vi "Vehicle Dynamics.vi"(9 "dt":sgl=1.0 format="%0.2f", 10 "Brake Force (N)":sgl, 11 "Transmission Output Torque (N-m)":sgl) -> (1 "Transmission Output Speed (rad/s)":sgl, 2 "Vehicle Speed (miles per hour)":sgl)   [LabVIEW 2016, in "NI-PCG Vehicle Model.lvlib"]
uses:
  NI-PCG Vehicle Model.lvlib
  Globals/Parameters.vi
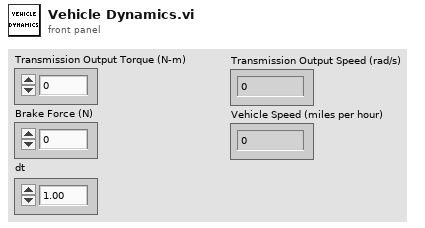
[diagram p1: front panel]
types:
  T1 = typedef "NI-PCG Vehicle Model.lvlib/Engine Parameters.ctl" = cluster{"Ambient Parameters":cluster{"Temperature (K)":sgl, "Pressure (Pa)":sgl}, "Air Parameters":cluster{"R (Ideal Gas Constant)":sgl, "Molecular Weight":sgl, "Cp (Specific Heat Constant)":sgl, "Density (kg/m^3)":sgl, "Stoichiometric A/F Ratio":sgl}, "Engine Geometry Parameters":cluster{"Cylinder Volume (l)":sgl, "J (Rotational Moment of Inertia)":sgl, "Minimuim Engine Speed":sgl, "Maximum Engine Speed":sgl, "Intake Manifold Volume (l)":sgl}, "Volumetric Efficiency Map":cluster{"MAP":sgl[], "RPM":sgl[], "Table":sgl[][]}, "Fuel LHV (J/kg)":sgl, "Combustion Efficiency Map":cluster{"Spark Timing (deg BTDC))":sgl[], "Engine Speed (RPM)":sgl[], "Combustion Efficiency":sgl[][]}, "Thermodynamic Efficiency":sgl}
  T2 = typedef "NI-PCG Vehicle Model.lvlib/Transmission Parameters.ctl" = cluster{"Final Drive Ratio":sgl, "Transmission Gear Ratios":cluster{"Gears":sgl[], "Gear Ratios":sgl[]}, "Torque Converter Map":cluster{"Speed Ratio":sgl[], "K Factor":sgl[], "Torque Ratio":sgl[]}, "Upshift Throttle":sgl[], "Downshift Throttle":sgl[], "Upshift Table":sgl[][], "Downshift Table":sgl[][], "Wait Time":u8}
  T3 = typedef "NI-PCG Vehicle Model.lvlib/Vehicle Parameters.ctl" = cluster{"Vehicle Mass (kg)":sgl, "Vehicle Cd":sgl, "Vehicle Frontal Area (m^2)":sgl, "Wheel Radius (m)":sgl, "Wheel Rolling Resistance":sgl}
  T4 = cluster{"Engine Parameters":T1, "Transmission Parameters":T2, "Vehicle Parameters":T3}
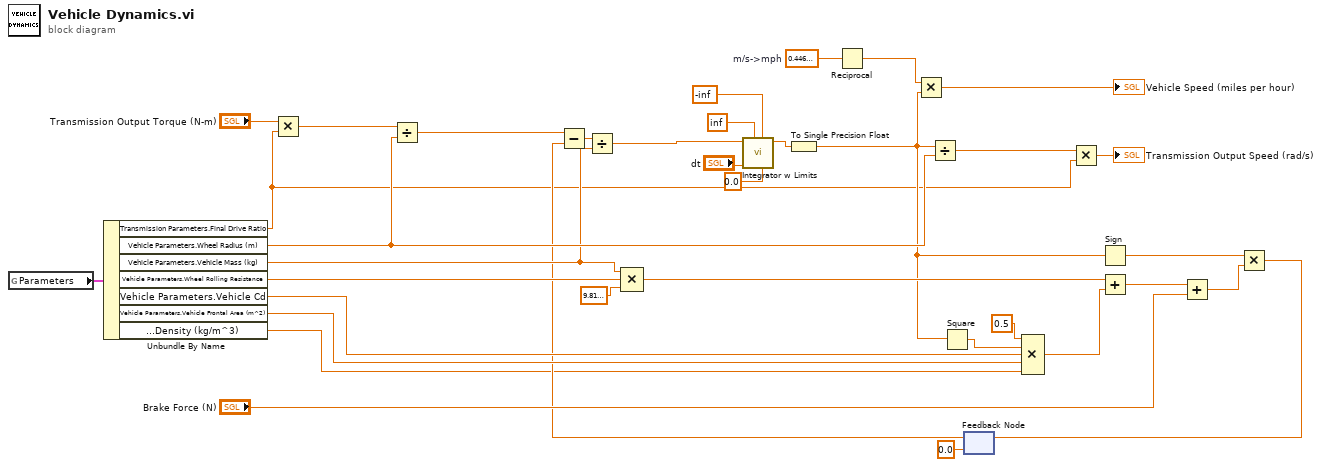
[diagram p0: block diagram]
diagram:
  w31 = sgl 0.447  # m/s->mph
  n1 = global read "Parameters.vi" "Parameters"() -> (w12:T4)
  n2 = Unbundle By Name(w12) -> ("Transmission Parameters.Final Drive Ratio"=w2:sgl, "Vehicle Parameters.Wheel Radius (m)"=w33:sgl, "Vehicle Parameters.Vehicle Mass (kg)"=w27:sgl, "Vehicle Parameters.Wheel Rolling Resistance"=w28:sgl, "Vehicle Parameters.Vehicle Cd"=w25:sgl, "Vehicle Parameters.Vehicle Frontal Area (m^2)"=w24:sgl, "Engine Parameters.Air Parameters.Density (kg/m^3)"=w1:sgl)
  n3 = Multiply(x="Transmission Output Torque (N-m)", y=w2) -> (x*y=w35:sgl)
  n4 = Divide(x=w35, y=w33) -> (x/y=w9:sgl)
  n5 = Compound Arithmetic op=MULTIPLY(w27, w28, sgl 9.81 ("value")) -> (w21:sgl)
  n6 = Reciprocal(x=w31) -> (1/x=w30:sgl)
  n7 = feedback #1(sgl 0.0) -> (w10:sgl)
  n8 = Subtract(x=w9, y=w10) -> (x-y=w34:sgl)
  n9 = Divide(x=w34, y=w27) -> (x/y=w4:sgl)
  n10 = call "Integrator w Limits.vi"("Initial Condition"=sgl 0.0, "lower limit"=sgl -inf, "upper limit"=sgl inf, "dt [s]"="dt", "x"=w4) -> ("Result"=w3:sgl)  [unwired: 6 in]
  n11 = To Single Precision Float(number=w3) -> (single precision float=w19:sgl)
  n12 = Multiply(x=w30, y=w19) -> (x*y=→"Vehicle Speed (miles per hour)":sgl)
  n13 = Divide(x=w19, y=w33) -> (x/y=w32:sgl)
  n14 = Square(x=w19) -> (x^2=w22:sgl)
  n15 = Compound Arithmetic op=MULTIPLY(sgl 0.5 ("value"), w22, w25, w24, w1) -> (w20:sgl)
  n16 = Multiply(x=w32, y=w2) -> (x*y=→"Transmission Output Speed (rad/s)":sgl)
  n17 = Sign(1:w19) -> (0:w16:sgl)
  n18 = Add(x=w21, y=w20) -> (x+y=w18:sgl)
  n19 = Add(x=w18, y="Brake Force (N)") -> (x+y=w15:sgl)
  n20 = Multiply(x=w16, y=w15) -> (x*y=w14:sgl)
  n21 = feedback-in #1(w14) -> ()
